vi "GetStatus.vi"(8 "error in (no error)":errorcluster, 10 "listener process":string, 11 "Qbus in":refnum<class "Qbus.lvclass">) -> (0 "error out":errorcluster, 1 "# pending insert":i32, 2 "# pending remove":i32, 3 "Qbus out":refnum<class "Qbus.lvclass">, 4 "# elements in queue":i32, 5 "max queue size":i32)   [LabVIEW 2017, in "Qbus.lvclass"]
uses:
  <vilib>/addons/Qbus/Qbus.lvclass
  <vilib>/addons/Qbus/Qbus.lvclass/Qbus.ctl
  <vilib>/addons/Qbus/controls/message.ctl
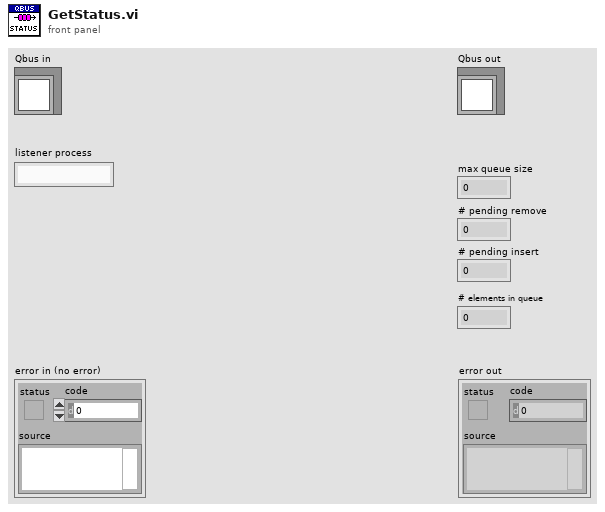
[diagram p1: front panel]
types:
  T1 = typedef "Qbus.lvclass/data.ctl" = cluster{"Queues":variant, "Subscriptions":variant, "MasterQ":string}
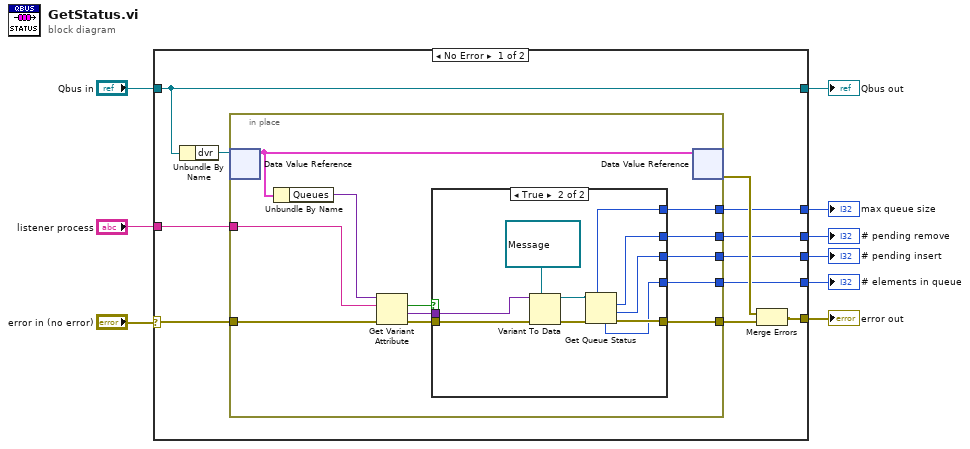
[diagram p0: block diagram]
diagram:
  n1 = case shown="No Error" "error in (no error)" {
    selector: "error in (no error)" -> [w16 w45]
    tunnel: [w17 w45] -> w8
    tunnel: [w14 w44] -> w6
    tunnel: "Qbus in" -> [w14 w44]
    tunnel: "listener process" -> [w15 _]
    tunnel: [w13 _] -> w4
    tunnel: [w12 _] -> w3
    tunnel: [w11 _] -> w2
    tunnel: [w10 _] -> w1
    frame No Error {
      n2 = Unbundle By Name(w14) -> ("dvr"=w18:refnum<data-value>)
      n3 = in-place {
        in-place-border: w16 -> [w30]
        in-place-border: [w31] -> w20
        in-place-border: w15 -> [w29]
        in-place-border: [w24] -> w13
        in-place-border: [w23] -> w12
        in-place-border: [w22] -> w11
        in-place-border: [w21] -> w10
        n4 = in-place-dvr #1(w18) -> (w32:T1)  [unwired: 1 out]
        n5 = Unbundle By Name(w32) -> ("Queues"=w28:variant)
        n6 = Get Variant Attribute(Variant=w28, name=w29, error in=w30) -> (found=w26:bool, value=w25:variant, error out=w27:errorcluster)  [unwired: 1 in, 1 out]
        n7 = case shown="True" w26 {
          tunnel: w27 -> [w33 w41]
          tunnel: [w33 w39] -> w31
          tunnel: w25 -> [_ w42]
          tunnel: [_ w37] -> w24
          tunnel: [_ w36] -> w23
          tunnel: [_ w35] -> w22
          tunnel: [_ w34] -> w21
          frame False {
          }
          frame True {
            n8 = Variant To Data(error in=w41, type=refnum<queue> refnum ("queue out"), Variant=w42) -> (data=w38:refnum<queue>, error out=w40:errorcluster)
            n9 = Get Queue Status(queue=w38, error in (no error)=w40) -> (max queue size=w37:i32, # pending remove=w36:i32, # pending insert=w35:i32, error out=w39:errorcluster, # elements in queue=w34:i32)  [unwired: 1 in, 3 out]
          }
        }
        n10 = in-place-dvr #1(w32) -> (w19:errorcluster)  [unwired: 1 out]
      }
      n11 = Merge Errors(w19, w20) -> (w17:errorcluster)
    }
    frame Error {
    }
  }
  "error out" <- w8
  "Qbus out" <- w6
  "max queue size" <- w4
  "# pending remove" <- w3
  "# pending insert" <- w2
  "# elements in queue" <- w1
